vi "ykgw_read.vi"(8 "error in (no error)":errorcluster, 11 "Instrument in":refnum<class "Instrument.lvclass">) -> (0 "error out":errorcluster, 2 "Data out":dbl[](array[numeric]), 3 "Instrument out":refnum<class "Instrument.lvclass">)   [LabVIEW 2019, in "Instrument.lvclass"]
uses:
  Instrument.lvclass
  Instrument.lvclass/Instrument.ctl
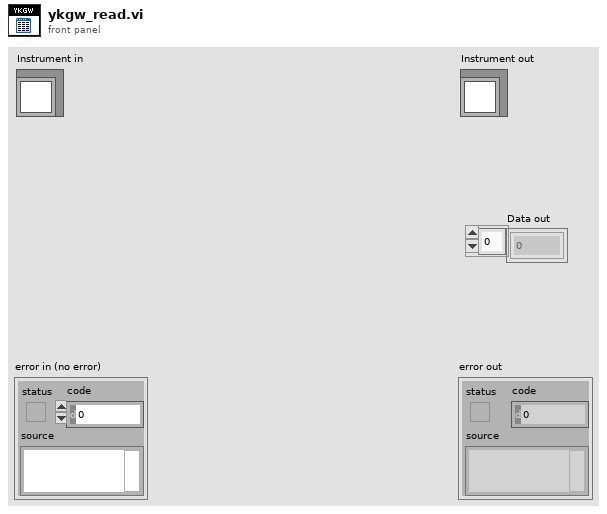
[diagram p1: front panel]
types:
  T1 = cluster{"Data[0]":dbl, "Data[1]":dbl, "Data[2]":dbl, "Data[3]":dbl, "Data[4]":dbl, "Data[5]":dbl, "Data[6]":dbl, "Data[7]":dbl, "Data[8]":dbl}
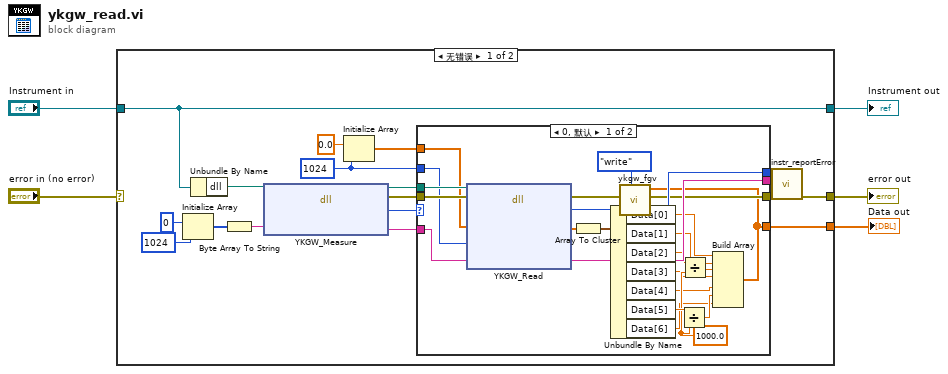
[diagram p0: block diagram]
diagram:
  n1 = case shown="无错误" "error in (no error)" {
    selector: "error in (no error)" -> [_ w52]
    tunnel: [w14 w52] -> w4
    tunnel: [w23 w51] -> w2
    tunnel: "Instrument in" -> [w23 w51]
    tunnel: [w9 _] -> w1
    frame No Error {
      w6 = 1024 ("dimension size")
      n2 = Initialize Array(u8 0 ("element"), 1024 ("dimension size")) -> (w11:u8[])
      n3 = Unbundle By Name(w23) -> ("dll"=w22:path)
      n4 = Byte Array To String(unsigned byte array=w11) -> (string=w10:string)
      n5 = dll-call lib="C:/Dev/22KW-Dyno/software/data/DynoAPI.dll" fn="YKGW_Measure"(path in=w22, "ErrorMsg"=w10) -> (path out=w21:path, error out=w20:errorcluster, "return type"=w18:i32, "ErrorMsg"=w19:string)  [unwired: 2 in]
      n6 = Initialize Array(0.0 ("element"), w6) -> (w8:dbl[])
      n7 = case shown="0, 默认" w18 {
        selector: w18 -> [_ w50]
        tunnel: w21 -> [w46 _]
        tunnel: w20 -> [w45 w49]
        tunnel: w19 -> [w44 w48]
        tunnel: [w38 w49] -> w17
        tunnel: [w43 w50] -> w16
        tunnel: [w42 w48] -> w15
        tunnel: [w28 w47] -> w9
        tunnel: w8 -> [w41 w47]
        tunnel: w6 -> [w40 _]
        frame 0, Default {
          w33 = 1000.0 ("y")
          n8 = dll-call lib="C:/Dev/22KW-Dyno/software/data/DynoAPI.dll" fn="YKGW_Read"(path in=w46, error in=w45, "Data"=w41, "NumSignal"=w40, "ErrorMsg"=w44) -> (error out=w39:errorcluster, "return type"=w43:i32, "Data"=w29:dbl[], "ErrorMsg"=w42:string)  [unwired: 2 in, 1 out]
          n9 = Array To Cluster(array=w29) -> (cluster=w36:T1)
          n10 = Unbundle By Name(w36) -> ("Data[0]"=w32:dbl, "Data[1]"=w31:dbl, "Data[2]"=w26:dbl, "Data[3]"=w30:dbl, "Data[4]"=w25:dbl, "Data[5]"=w35:dbl, "Data[6]"=w24:dbl)
          n11 = Divide(x=w35, y=w33) -> (x/y=w34:dbl)
          n12 = Divide(x=w26, y=w33) -> (x/y=w27:dbl)
          n13 = Build Array(w32, w31, w27, w30, w25, w34, w24) -> (w28:dbl[])
          n14 = call "ykgw_fgv.vi"("mode"=enum16{"read", "write"}."write", "error in (no error)"=w39, "Data in"=w28) -> ("error out"=w38:errorcluster)  [unwired: 4 in, 4 out]
        }
        frame ..-1 {
        }
      }
      n15 = call "instr_reportError.vi"("error in (no error)"=w17, "errorMsg"=w15, "return type"=w16) -> ("error out"=w14:errorcluster)  [unwired: 8 in]
    }
    frame Error {
    }
  }
  "error out" <- w4
  "Instrument out" <- w2
  "Data out" <- w1
